vi "createqueue.vi"(2 "error in (no error)":errorcluster) -> (0 "error out":errorcluster, 1 "queue out":T1)   [LabVIEW 2011]
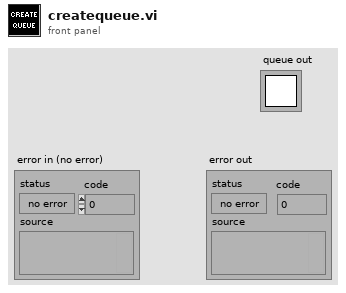
[diagram p1: front panel]
types:
  T1 = typedef "Queue RefNum" = refnum<k1>
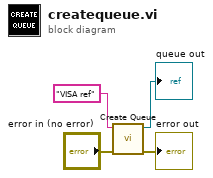
[diagram p0: block diagram]
diagram:
  n1 = call <vilib>:"Create Queue.vi"("error in (no error)"="error in (no error)", "name (unnamed)"="VISA ref") -> ("error out"=→"error out":errorcluster, "queue out"=→"queue out":T1)  [unwired: 3 in, 1 out]
